vi "Compute_RectAverage_Poly.vi"   [LabVIEW 2012]
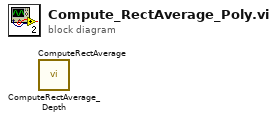
[diagram p0: block diagram]
diagram:
  n1 = call "ComputeRectAverage_Depth.vi"() -> ()  [unwired: 5 in, 2 out]
  n2 = call "ComputeRectAverage.vi"() -> ()  [unwired: 3 in, 4 out]
